vi "my1.vi"() -> ()   [LabVIEW 2015]
uses:
  <vilib>/NXT/Block Support/NXT_InputPort.ctl
  <vilib>/NXT/Block Support/NXT_OutputPort.ctl
  <vilib>/NXT/Dual Mode Library/Sensors/Sonar_cm.vi
  <vilib>/NXT/Dual Mode Library/Sensors/Light_On.vi
  <vilib>/NXT/Dual Mode Library/Sensors/Touch_Pressed.vi
  <vilib>/NXT/NXTIO Xnodes/NXTIONodeSubVIs/LEGOMoveAllMotors.vi
  <vilib>/NXT/NXTIO Xnodes/NXTIONodeSubVIs/NXTMoveMotors.vi
  <vilib>/NXT/Dual Mode Library/Waits/Wait_Num.vi
  <vilib>/NXT/NXTIO Xnodes/AddressXNode/NXTIOAddress.xnode
  <vilib>/NXT/Subs/LVHSConnector.ctl
  <vilib>/NXT/NXTIO Xnodes/NXTIOXNode/NXTIO.xnode
  <vilib>/NXT/LegoClasses/BrickReference/BrickReference.lvclass
panel:
  out "Yes / No 2":bool
  out "Yes / No":bool
  in  "stop":bool
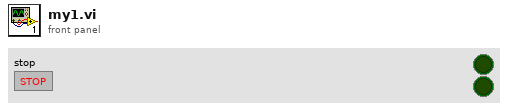
[diagram p1: front panel]
types:
  T1 = typedef "NXT_InputPort.ctl" = u32
  T2 = typedef "NXT_OutputPort.ctl" = u8
  T3 = typedef "LVHSConnector.ctl" = refnum<class "BrickReference.lvclass">
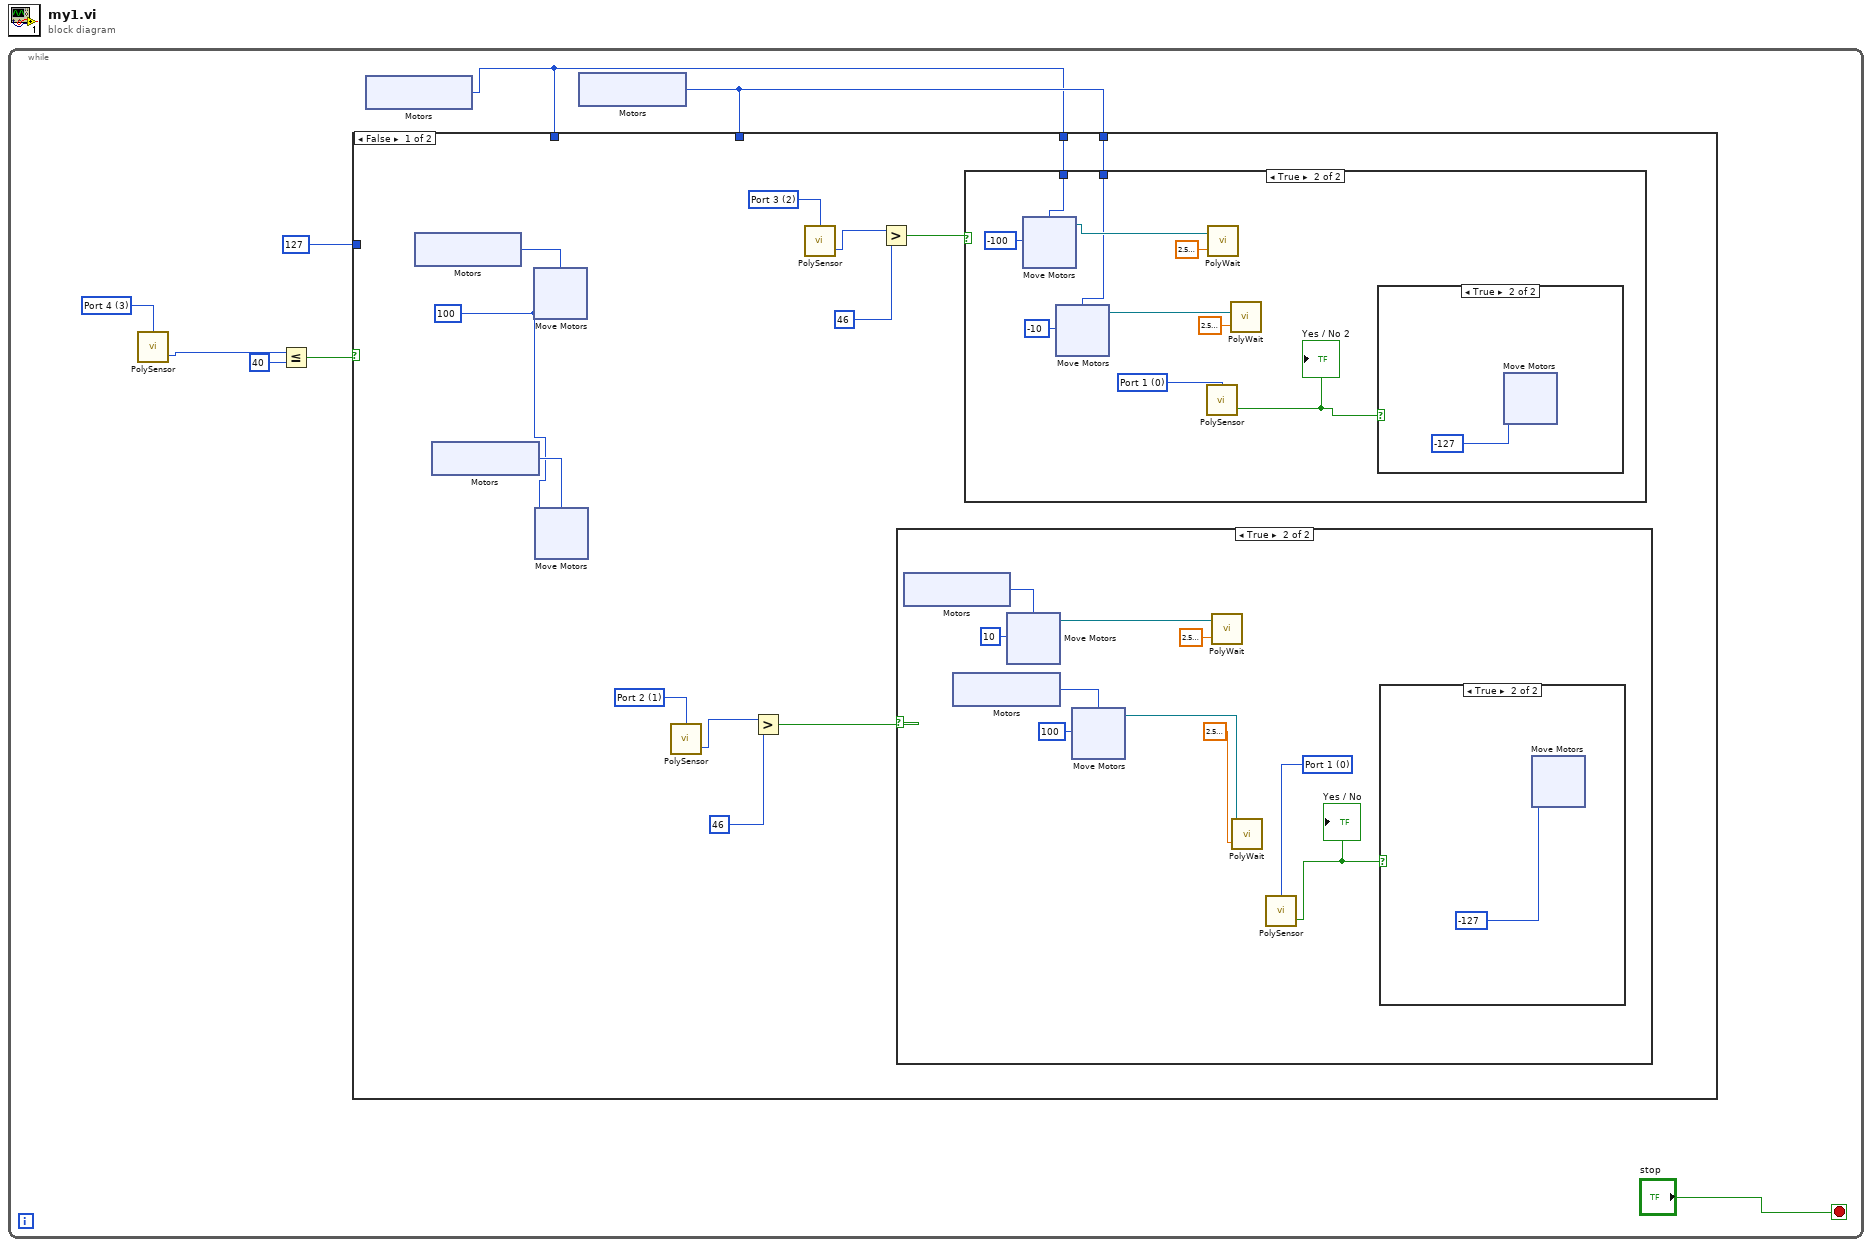
[diagram p0: block diagram]
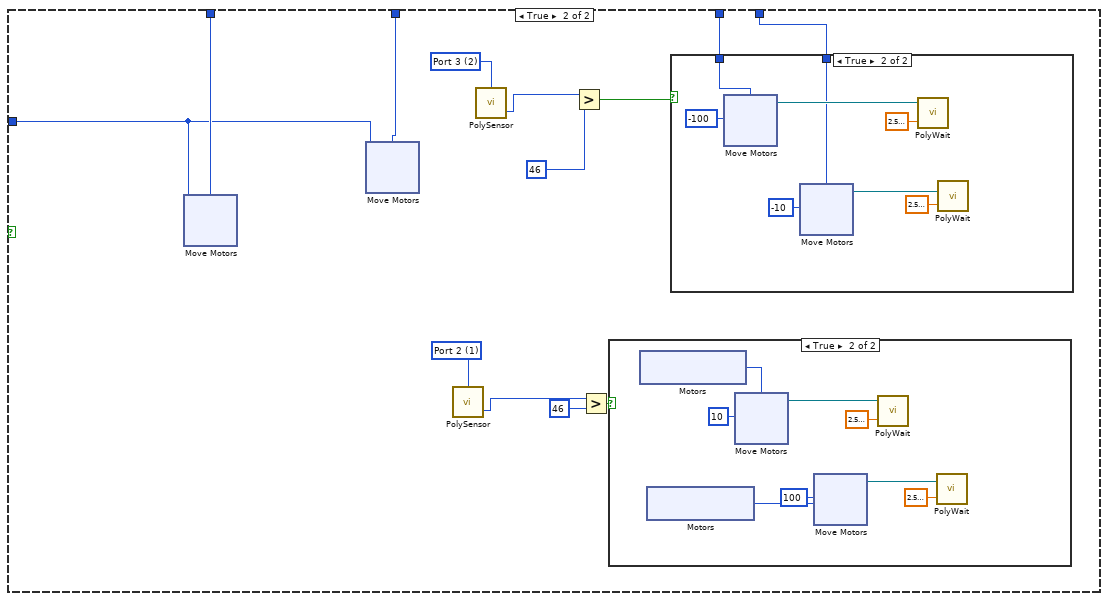
[diagram p6: hidden frame]
diagram:
  n1 = while {
    stop <- "stop" stop-if-true
    w8 = T1 3 items=["Port 1", "Port 2", "Port 3", "Port 4"] ("Port (Port 4)")
    n2 = call-poly <vilib>:"PolySensor.vi"("Port (Port 4)"=w8) -> ("Distance (cm)"=w7:i16)  [unwired: 2 in, 1 out]
    n3 = Less Or Equal?(x=w7, y=i16 40) -> (x <= y?=w5:bool)
    n4 = xnode "Motors"() -> ("Motor"=w2:T2)
    n5 = xnode "Motors"() -> ("Motor"=w3:T2)
    n6 = case shown="False" w5 {
      tunnel: w2 -> [_ w118]
      tunnel: w3 -> [_ w117]
      tunnel: i8 127 ("Power/Speed 1") -> [_ w116]
      tunnel: w3 -> [w11 w110]
      tunnel: w2 -> [w12 w111]
      frame False {
        w13 = T1 1 items=["Port 1", "Port 2", "Port 3", "Port 4"] ("Port (Port 3)")
        w20 = T1 2 items=["Port 1", "Port 2", "Port 3", "Port 4"] ("Port (Port 3)")
        w21 = i8 100 ("Power/Speed 1")
        n7 = xnode "Motors"() -> ("Motor"=w23:T2)
        n8 = xnode "Motors"() -> ("Motor"=w22:T2)
        n9 = xnode "Move Motors"("Power/Speed 1"=w21, "Motors"=w23) -> ()  [unwired: 1 in, 1 out]
        n10 = xnode "Move Motors"("Power/Speed 1"=w21, "Motors"=w22) -> ()  [unwired: 1 in, 1 out]
        n11 = call-poly <vilib>:"PolySensor.vi"("Port (Port 3)"=w13) -> ("Scaled Value"=w15:i16)  [unwired: 2 in, 1 out]
        n12 = Greater?(x=w15, y=i16 46) -> (0:w16:bool)
        n13 = call-poly <vilib>:"PolySensor.vi"("Port (Port 3)"=w20) -> ("Scaled Value"=w18:i16)  [unwired: 2 in, 1 out]
        n14 = Greater?(x=w18, y=i16 46) -> (0:w19:bool)
        n15 = case shown="True" w16 {
          frame False {
          }
          frame True {
            w25 = T1 0 items=["Port 1", "Port 2", "Port 3", "Port 4"] ("Port (Port 1)")
            n16 = xnode "Motors"() -> ("Motor"=w31:T2)
            n17 = xnode "Motors"() -> ("Motor"=w30:T2)
            n18 = xnode "Move Motors"("Power/Speed 1"=i8 10, "Motors"=w31) -> ("NXT/EV3"=w33:T3)  [unwired: 1 in]
            n19 = xnode "Move Motors"("Power/Speed 1"=i8 100, "Motors"=w30) -> ("NXT/EV3"=w32:T3)  [unwired: 1 in]
            n20 = call-poly <vilib>:"PolyWait.vi"("Time (1 sec)"=sgl 2.6, "NXT/EV3"=w33) -> ()  [unwired: 2 in, 1 out]
            n21 = call-poly <vilib>:"PolyWait.vi"("Time (1 sec)"=sgl 2.6, "NXT/EV3"=w32) -> ()  [unwired: 2 in, 1 out]
            n22 = call-poly <vilib>:"PolySensor.vi"("Port (Port 1)"=w25) -> ("Yes / No"=w24:bool)  [unwired: 2 in, 1 out]
            "Yes / No" <- w24
            n23 = case shown="True" w24 {
              frame False {
              }
              frame True {
                n24 = xnode "Move Motors"("Power/Speed 1"=i8 -127 ("Power/Speed 2")) -> ()  [unwired: 2 in, 1 out]
              }
            }
          }
        }
        n25 = case shown="True" w19 {
          tunnel: w12 -> [_ w65]
          tunnel: w11 -> [_ w64]
          frame False {
          }
          frame True {
            w59 = T1 0 items=["Port 1", "Port 2", "Port 3", "Port 4"] ("Port (Port 1)")
            n26 = xnode "Move Motors"("Power/Speed 1"=i8 -100, "Motors"=w65) -> ("NXT/EV3"=w67:T3)  [unwired: 1 in]
            n27 = xnode "Move Motors"("Power/Speed 1"=i8 -10, "Motors"=w64) -> ("NXT/EV3"=w66:T3)  [unwired: 1 in]
            n28 = call-poly <vilib>:"PolySensor.vi"("Port (Port 1)"=w59) -> ("Yes / No"=w58:bool)  [unwired: 2 in, 1 out]
            "Yes / No 2" <- w58
            n29 = call-poly <vilib>:"PolyWait.vi"("Time (1 sec)"=sgl 2.6, "NXT/EV3"=w67) -> ()  [unwired: 2 in, 1 out]
            n30 = call-poly <vilib>:"PolyWait.vi"("Time (1 sec)"=sgl 2.6, "NXT/EV3"=w66) -> ()  [unwired: 2 in, 1 out]
            n31 = case shown="True" w58 {
              frame False {
              }
              frame True {
                n32 = xnode "Move Motors"("Power/Speed 1"=i8 -127 ("Power/Speed 2")) -> ()  [unwired: 2 in, 1 out]
              }
            }
          }
        }
      }
      frame True {
        w109 = T1 1 items=["Port 1", "Port 2", "Port 3", "Port 4"] ("Port (Port 3)")
        w112 = T1 2 items=["Port 1", "Port 2", "Port 3", "Port 4"] ("Port (Port 3)")
        n33 = xnode "Move Motors"("Power/Speed 1"=w116, "Motors"=w118) -> ()  [unwired: 1 in, 1 out]
        n34 = xnode "Move Motors"("Power/Speed 1"=w116, "Motors"=w117) -> ()  [unwired: 1 in, 1 out]
        n35 = call-poly <vilib>:"PolySensor.vi"("Port (Port 3)"=w109) -> ("Scaled Value"=w107:i16)  [unwired: 2 in, 1 out]
        n36 = call-poly <vilib>:"PolySensor.vi"("Port (Port 3)"=w112) -> ("Scaled Value"=w115:i16)  [unwired: 2 in, 1 out]
        n37 = Greater?(x=w115, y=i16 46) -> (0:w113:bool)
        n38 = Greater?(x=w107, y=i16 46) -> (0:w108:bool)
        n39 = case shown="True" w108 {
          frame False {
          }
          frame True {
            n40 = xnode "Motors"() -> ("Motor"=w126:T2)
            n41 = xnode "Motors"() -> ("Motor"=w125:T2)
            n42 = xnode "Move Motors"("Power/Speed 1"=i8 10, "Motors"=w126) -> ("NXT/EV3"=w124:T3)  [unwired: 1 in]
            n43 = xnode "Move Motors"("Power/Speed 1"=i8 100, "Motors"=w125) -> ("NXT/EV3"=w123:T3)  [unwired: 1 in]
            n44 = call-poly <vilib>:"PolyWait.vi"("Time (1 sec)"=sgl 2.6, "NXT/EV3"=w124) -> ()  [unwired: 2 in, 1 out]
            n45 = call-poly <vilib>:"PolyWait.vi"("Time (1 sec)"=sgl 2.6, "NXT/EV3"=w123) -> ()  [unwired: 2 in, 1 out]
          }
        }
        n46 = case shown="True" w113 {
          tunnel: w111 -> [_ w148]
          tunnel: w110 -> [_ w147]
          frame False {
          }
          frame True {
            n47 = xnode "Move Motors"("Power/Speed 1"=i8 -100, "Motors"=w148) -> ("NXT/EV3"=w149:T3)  [unwired: 1 in]
            n48 = xnode "Move Motors"("Power/Speed 1"=i8 -10, "Motors"=w147) -> ("NXT/EV3"=w150:T3)  [unwired: 1 in]
            n49 = call-poly <vilib>:"PolyWait.vi"("Time (1 sec)"=sgl 2.6, "NXT/EV3"=w149) -> ()  [unwired: 2 in, 1 out]
            n50 = call-poly <vilib>:"PolyWait.vi"("Time (1 sec)"=sgl 2.6, "NXT/EV3"=w150) -> ()  [unwired: 2 in, 1 out]
          }
        }
      }
    }
  }
